vi "JKISM++ Mark As Worker Module.vi"(9 "JKISM Name":string) -> (2 "JKISM Name(marked as worker)":string)   [LabVIEW 2014, in "JKI State Machine++.lvlib"]
doc: "Append '#' to JKISM Name, to mark this module is a worker, who shares the same message queue with workers with the same name. A real name with uuid generated will be assigned to this JKISM module.\n\n<b>Inputs:</b>\n - <b>JKISM Name</b>: JKISM module name.\n\n<b>Outputs:</b>\n - <b>JKISM Name(marked as worker)</b>: JKISM module name with '#' appended."
uses:
  JKI State Machine++.lvlib
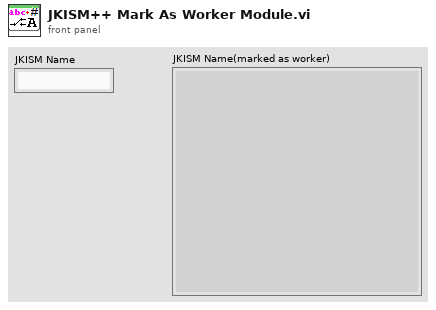
[diagram p1: front panel]
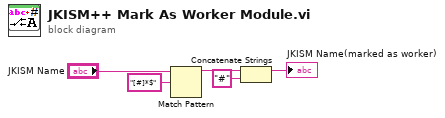
[diagram p0: block diagram]
diagram:
  n1 = Match Pattern(string="JKISM Name", regular expression="[#]*$") -> (before substring=w3:string)  [unwired: 1 in, 3 out]
  n2 = Concatenate Strings(w3, "#" ("string")) -> (→"JKISM Name(marked as worker)":string)
